vi "Read Transfer Groups State Data.vi"(8 "error in (no error)":errorcluster, 11 "Framework Status in":refnum<class "Framework Status.lvclass">) -> (0 "error out":errorcluster, 2 "transfer groups state data":T1[](array[typedef]) {"duration" format="%d us"}, 3 "Framework Status out":refnum<class "Framework Status.lvclass">)   [LabVIEW 2017, in "DSF Core.lvlib" / "Framework Status.lvclass"]
uses:
  Framework Status.lvclass
  Status/Status Data.ctl
  Framework Status.lvclass/Framework Status.ctl
  Status/Status Pointer.lvclass
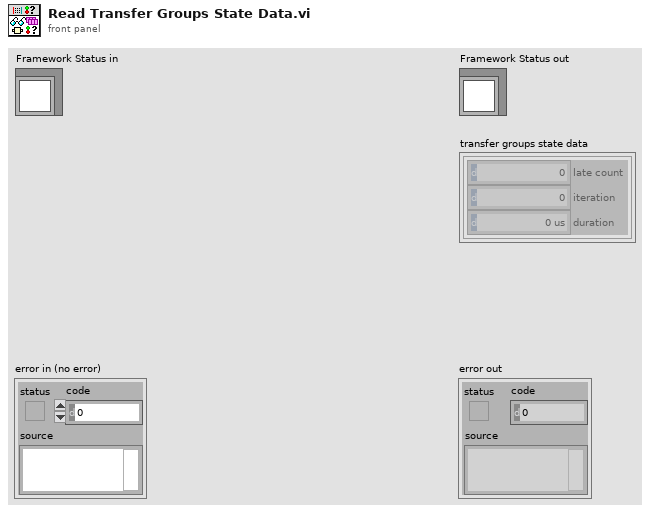
[diagram p1: front panel]
types:
  T1 = typedef "DSF Core.lvlib/Status Pointer.lvclass/Status Data.ctl" = cluster{"late count":u64, "iteration":u64, "duration":u32}
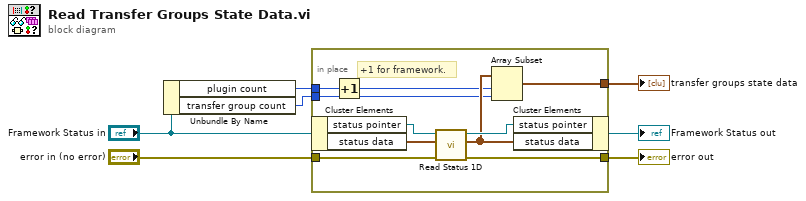
[diagram p0: block diagram]
diagram:
  n1 = Unbundle By Name("Framework Status in") -> ("plugin count"=w2:i32, "transfer group count"=w1:i32)
  n2 = in-place {
    in-place-border: "error in (no error)" -> [w14]
    in-place-border: [w13] -> w5
    in-place-border: [w12] -> w4
    in-place-border: w2 -> [w10]
    in-place-border: w1 -> [w8]
    # "+1 for framework."
    n3 = in-place-cluster #1("Framework Status in") -> ("status pointer"=w17:refnum<class "Status Pointer.lvclass">, "status data"=w16:T1[])
    n4 = Increment(x=w10) -> (x+1=w9:i32)
    n5 = call "Read Status 1D.vi"("error in (no error)"=w14, "statuses in"=w16, "status pointer in"=w17) -> ("error out"=w13:errorcluster, "statuses out"=w11:T1[], "status pointer out"=w15:refnum<class "Status Pointer.lvclass">)  [unwired: 6 in]
    n6 = Array Subset(array=w11, index=w9, length=w8) -> (w12:T1[])
    n7 = in-place-cluster #1("status pointer"=w15, "status data"=w11) -> (→"Framework Status out":refnum<class "Framework Status.lvclass">)
  }
  "error out" <- w5
  "transfer groups state data" <- w4
